vi "Confocal_0919 (1).vi"() -> ()   [LabVIEW 2017]
uses:
  <vilib>/Math Plots/2D Math Plots/XY Plot Matrix/XY Plot Matrix XCtrl/XY Plot Matrix.xctl
  Public/Documents/SIToolkit/LabVIEW/ExamplesXX_4_3_1_4/Spectroscopy Applications/GlobalCamOpen.vi
  Public/Documents/SIToolkit/LabVIEW/ExamplesXX_4_3_1_4/Spectroscopy Applications/GlobalInitializeFlag.vi
  Public/Documents/SIToolkit/LabVIEW/ExamplesXX_4_3_1_4/Spectroscopy Applications/GlobalTimingMode.vi
  Public/Documents/SIToolkit/LabVIEW/ExamplesXX_4_3_1_4/Spectroscopy Applications/GlobalFramesToStr.vi
  Public/Documents/SIToolkit/LabVIEW/ExamplesXX_4_3_1_4/Spectroscopy Applications/GlobalAcquireFocusFlag.vi
  Public/Documents/SIToolkit/LabVIEW/ExamplesXX_4_3_1_4/Spectroscopy Applications/GlobalExposure.vi
  <vilib>/Math Plots/2D Math Plots/XY Plot Matrix/XY Plot Matrix Datatype/XY Plot Matrix Datatype.lvclass
panel:
  out "Position 7":dbl[](array[numeric]) format="%.6f"
  out "Position 4":dbl[](array[numeric]) format="%.6f"
  in  "error PI Stage":errorcluster
  out "error out 2":errorcluster
  in  "Tab Control":T1(tab)
  in  "Focus/Acquire Mode":u32=1 min=1 max=5 step=1
  in  "Number of Frames to store":u32=1 min=1 step=1
  in  "Timing Mode":u32(ring)=1 items=["N/A", "Free Run/Timed", "Trigger First (PM only)", "Ext Sync/Strobed ", "Variable Exp (PM only)", "Flash Mode (PM only)"]
  out "Pixel Time":i32
  out "Bit Depth":i32
  out "ReadOut port":i32
  out "ADC Speed":i32
  in  "Set Experiment \nParameters, Initialize \nCamera/Controller":bool
  out "Read Temp.":dbl format="%.2f"
  in  "Set Temp.":dbl format="%.2f"
  in  "Exposure 2":dbl=0.2 format="%.2f"
  out "Controller Initialized":bool
  in  "error in":errorcluster
  out "error out":errorcluster
  in  "Power":dbl=10.0
  in  "Frequency":dbl=2810.0
  in  "Release Camera":bool
  out "Position 6":dbl[](array[numeric]) format="%.6f"
  out "Conn. Axis 5":string[](array[string])
  out "error out 3":errorcluster
  in  "stop":bool
  out "Read Frequency":dbl
  in  "Initial Frequency":dbl=2820.0
  in  "Final Frequency":dbl=2890.0
  in  "Step Size":dbl=3.0
  in  "OK Button 3":bool
  out "XY Plot Matrix":refnum<class "XY Plot Matrix Datatype.lvclass">[](xcontrol)
  out "history":dbl[][](array[numeric])
  in  "Number of Scans":i32
  out "COM Error":bool
  out "Camera Opened":bool
  out "Scan":i32
  in  "Number of Steps Left":dbl=5.0 format="%#_13g"
  in  "OK Button 5":bool
  in  "Step Size (microns)":dbl[](array[numeric])=[0.01]
  out "XY Plot Matrix":refnum<class "XY Plot Matrix Datatype.lvclass">[](xcontrol)
  in  "Number of Steps Down":dbl=5.0 format="%#_13g"
  out "Position":dbl[](array[numeric]) format="%.6f"
  out "Position 3":dbl[](array[numeric]) format="%.6f"
  in  "stop 2":bool
  out "Line Number":i32
  out "Position 2":dbl[](array[numeric]) format="%.6f"
  in  "?":bool
  out "Position 5":dbl[](array[numeric]) format="%.6f"
  in  "Step Size (microns) Y":dbl[](array[numeric])=[0.01]
  in  "Step Size (microns) X":dbl[](array[numeric])=[0.01]
  out "Position 8":dbl[](array[numeric]) format="%.6f"
  in  "?":bool
  in  "OK Button 4":bool
  in  "Frequency":dbl=2820.0
  out "XY Plot Matrix 2":refnum<class "XY Plot Matrix Datatype.lvclass">[](xcontrol) caption="XY Plot Matrix"
  out "history 2":dbl[][](array[numeric])
  in  "Points":i32=40
  in  "number of scans":i32=20
  out "Scan #":i32
  out "Point #":i32
  out "Acquire Graph":sgl[](graph)
  out "Collecting Data":bool
  in  "Full File Name for Acqure":path
  in  "OK Button":bool
  # "The following are read \nfrom camera after setting\nvalues to left.\n-1 value means item is not \nsupported by camera."
  # "Stage position on connection."
  # "Be sure to put in a full file name below before starting."
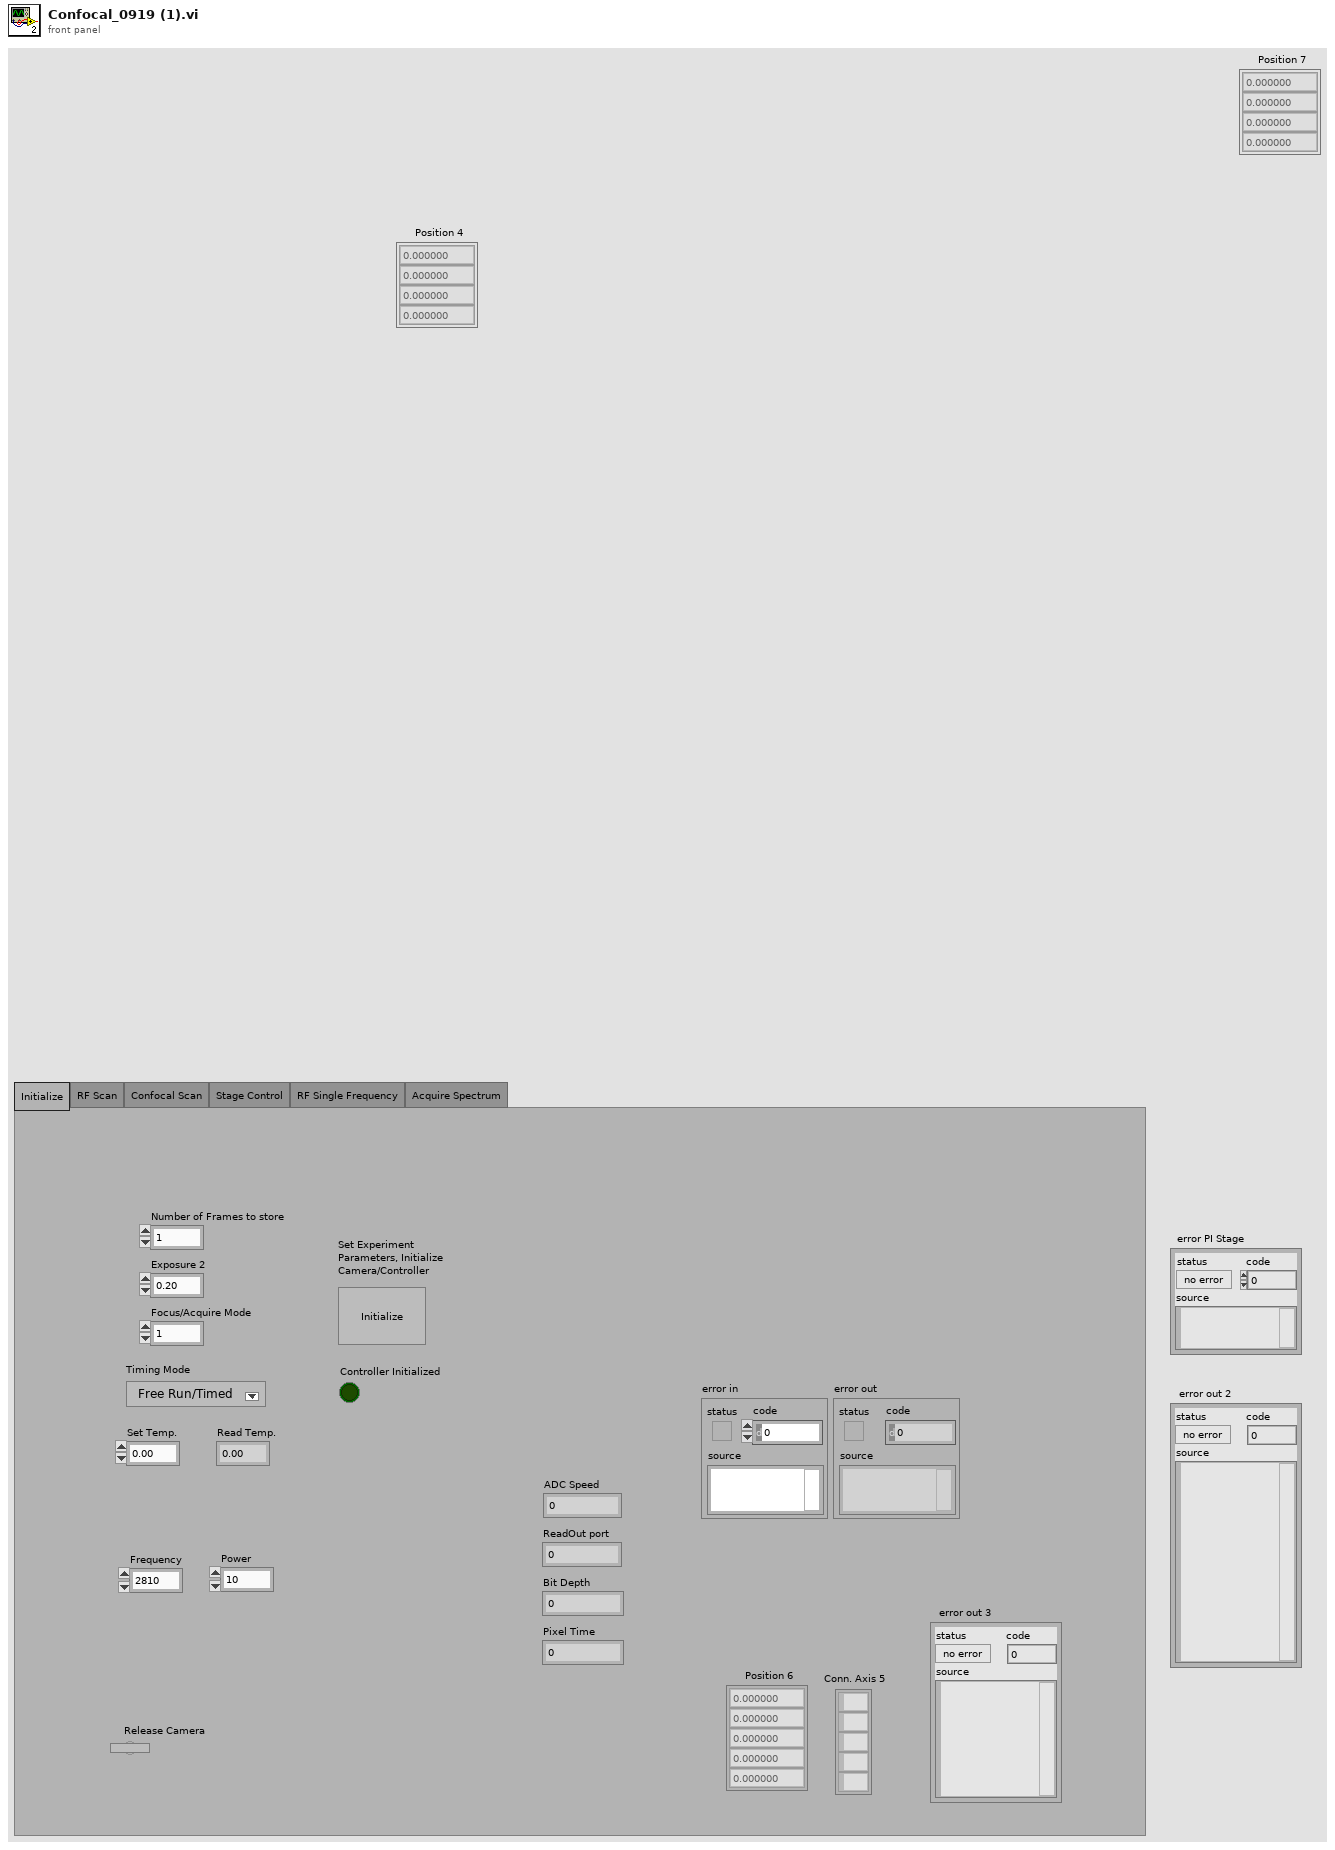
[diagram p1: front panel]
types:
  T1 = enum32{"Initialize", "RF Scan", "Confocal Scan", "Stage Control", "RF Single Frequency", "Acquire Spectrum"}
  T2 = cluster{"X start":u32, "X end":u32, "X Binning/Grouping":u32, "Y start":u32, "Y end":u32, "Y Binning/Grouping":u32}
  T3 = cluster{"Host address/name":string, "Port":i32, "Board":i32, "TCP/IP Search?":bool}
  T4 = cluster{"Camera Handle":u32, "Pulser Handle":u32, "File Handle":u32, "Display Handle":u32, "Image Handle":u32}
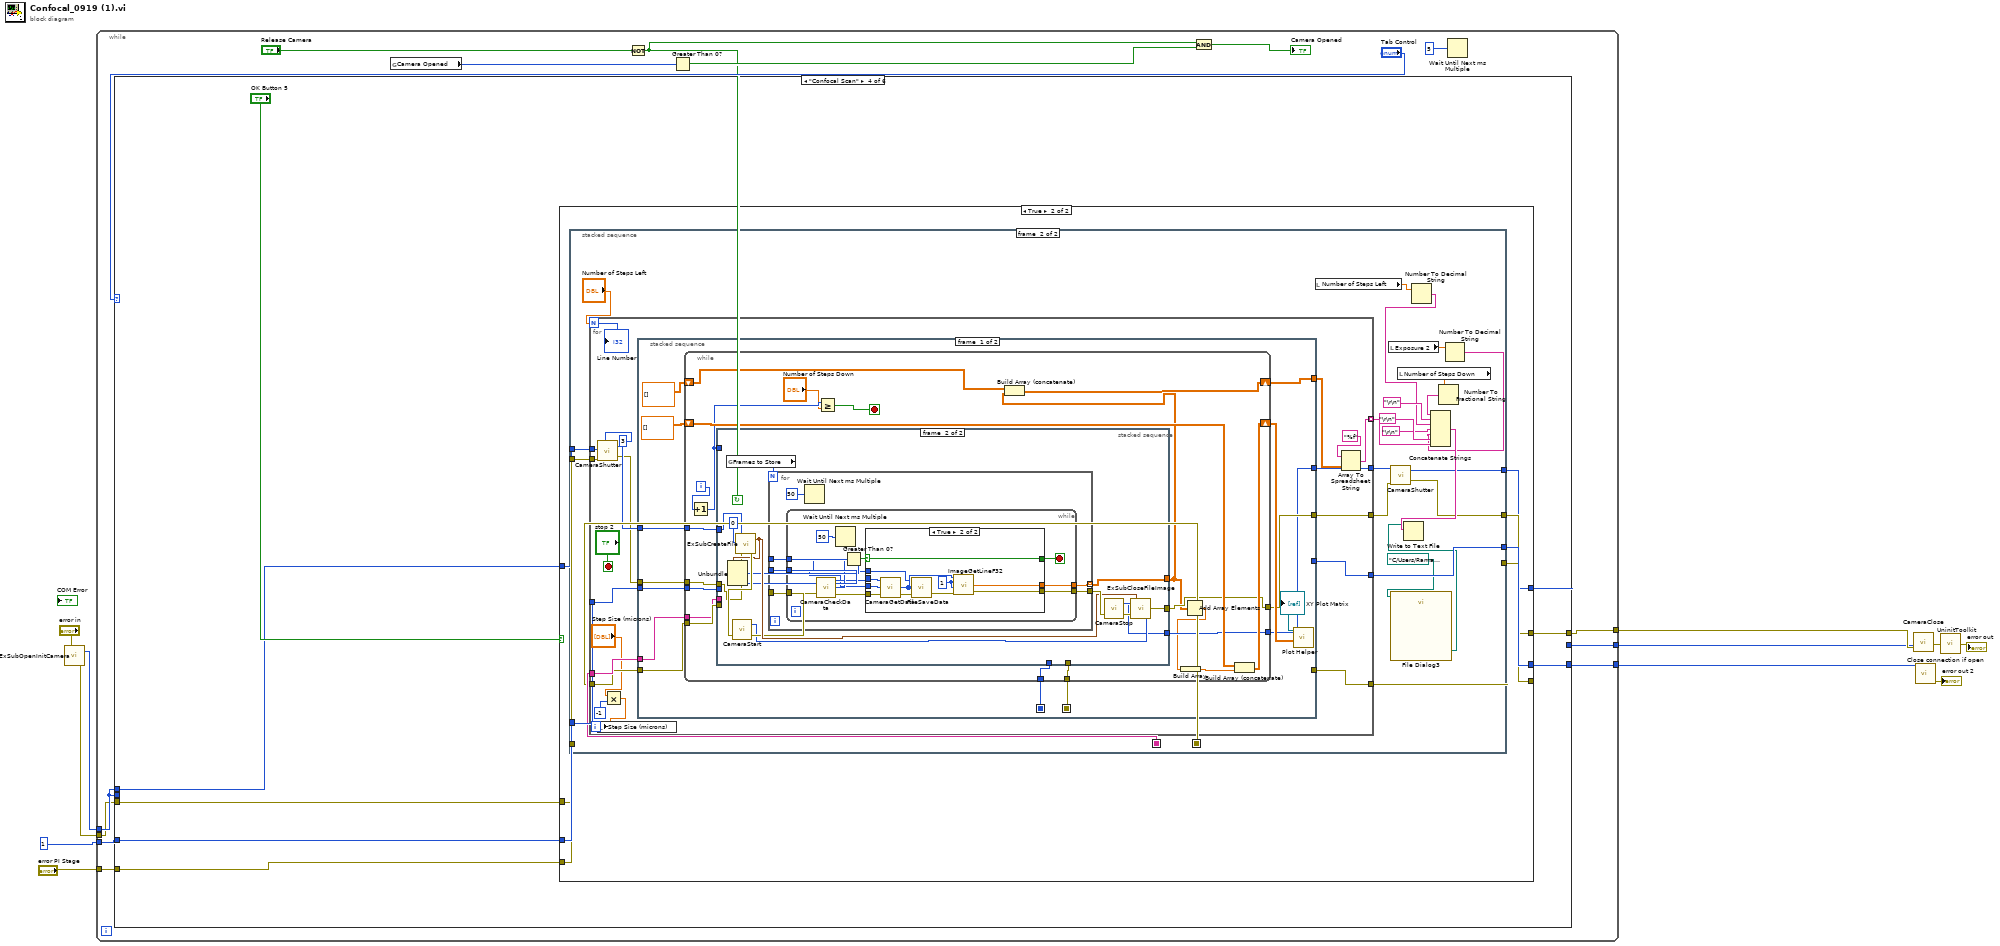
[diagram p0: block diagram]
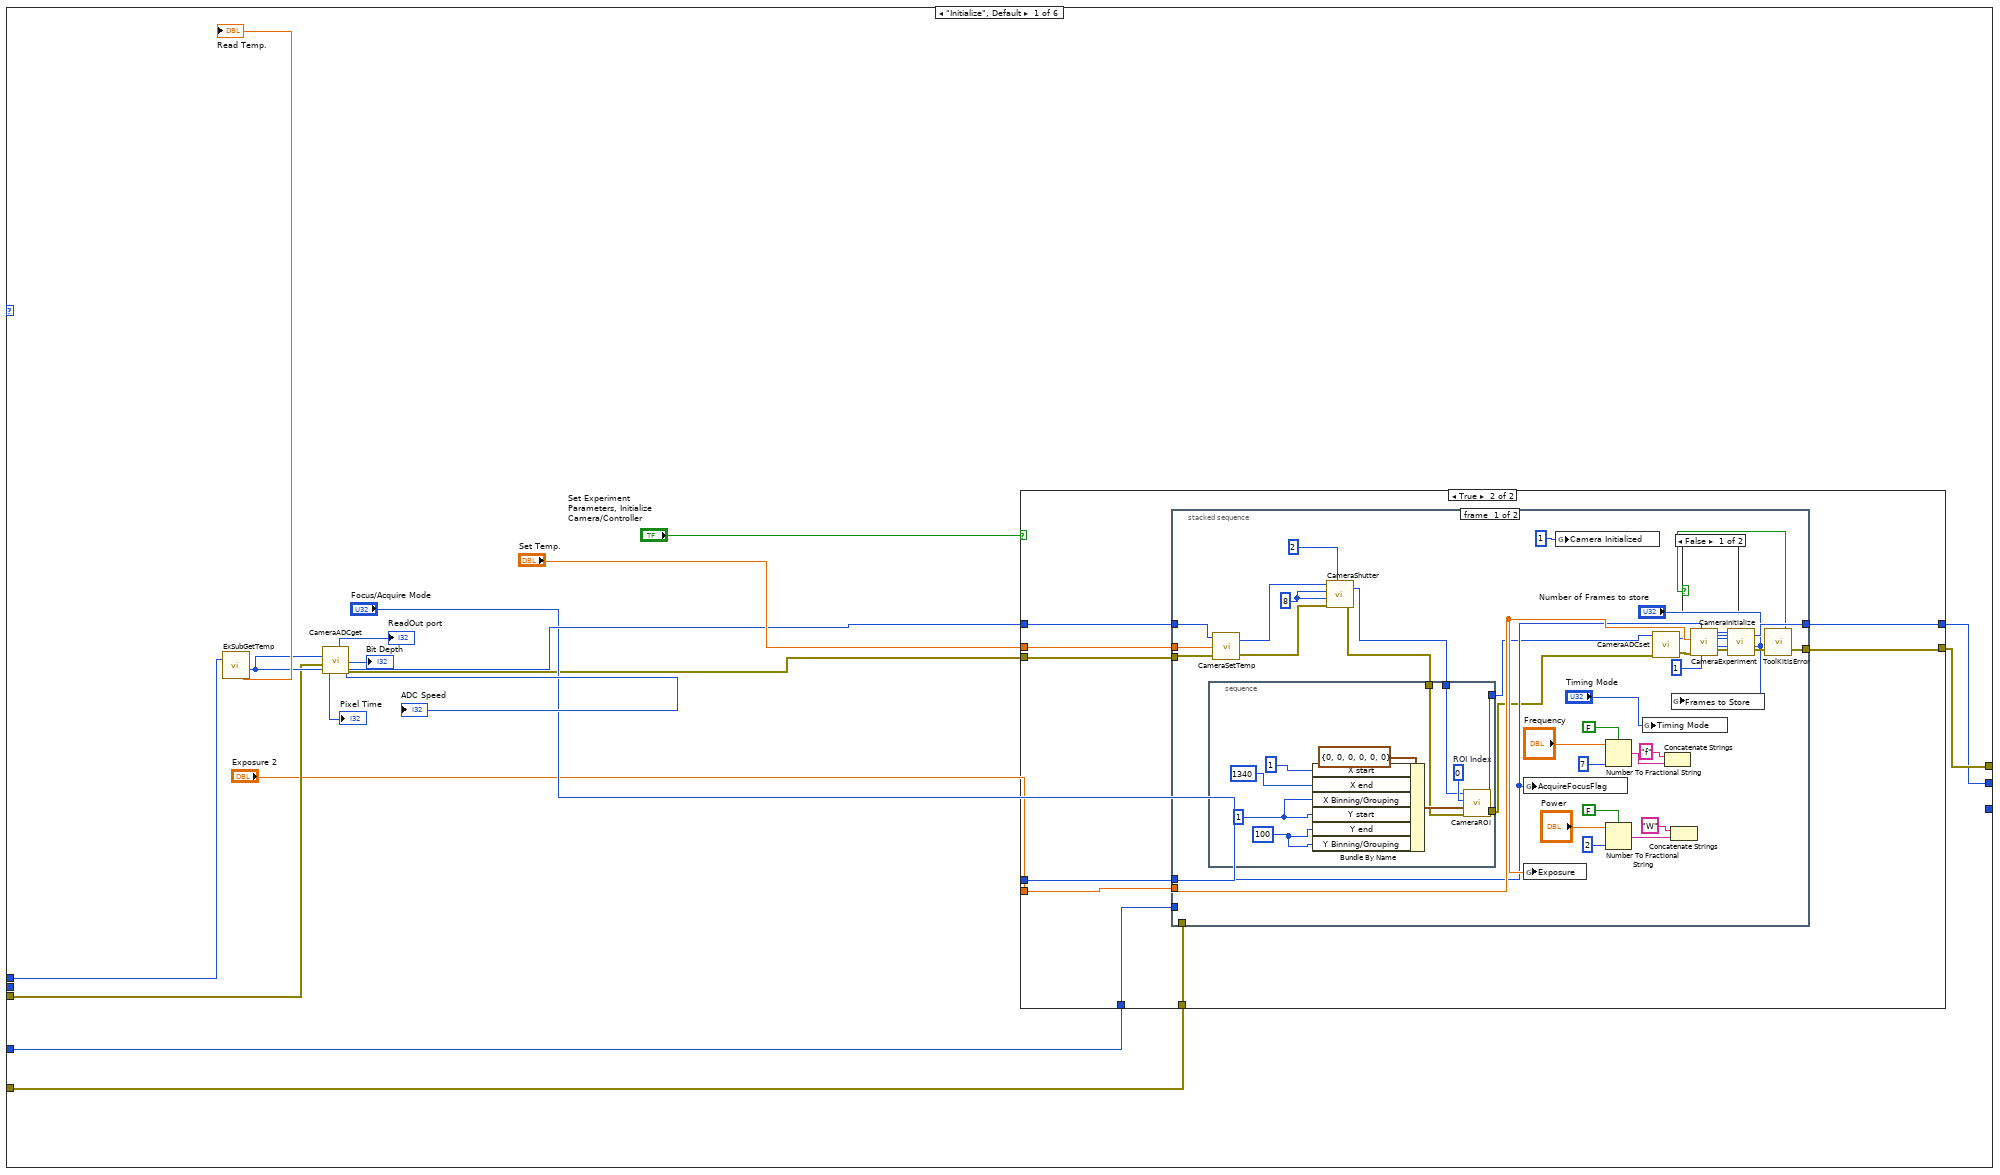
[diagram p2: hidden frame]
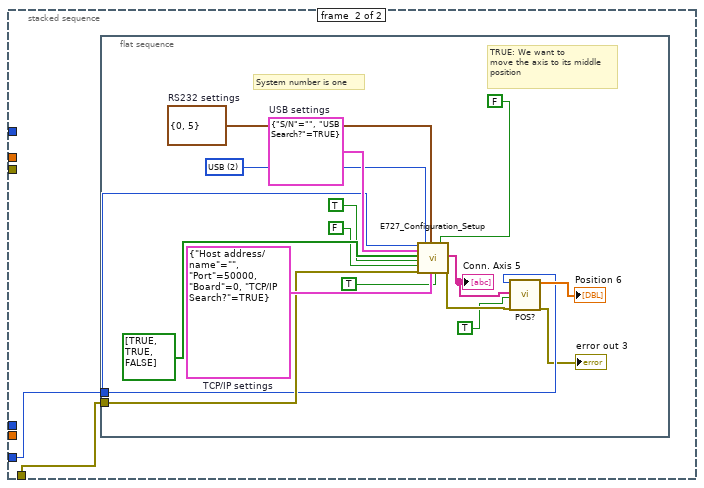
[diagram p5: hidden frame]
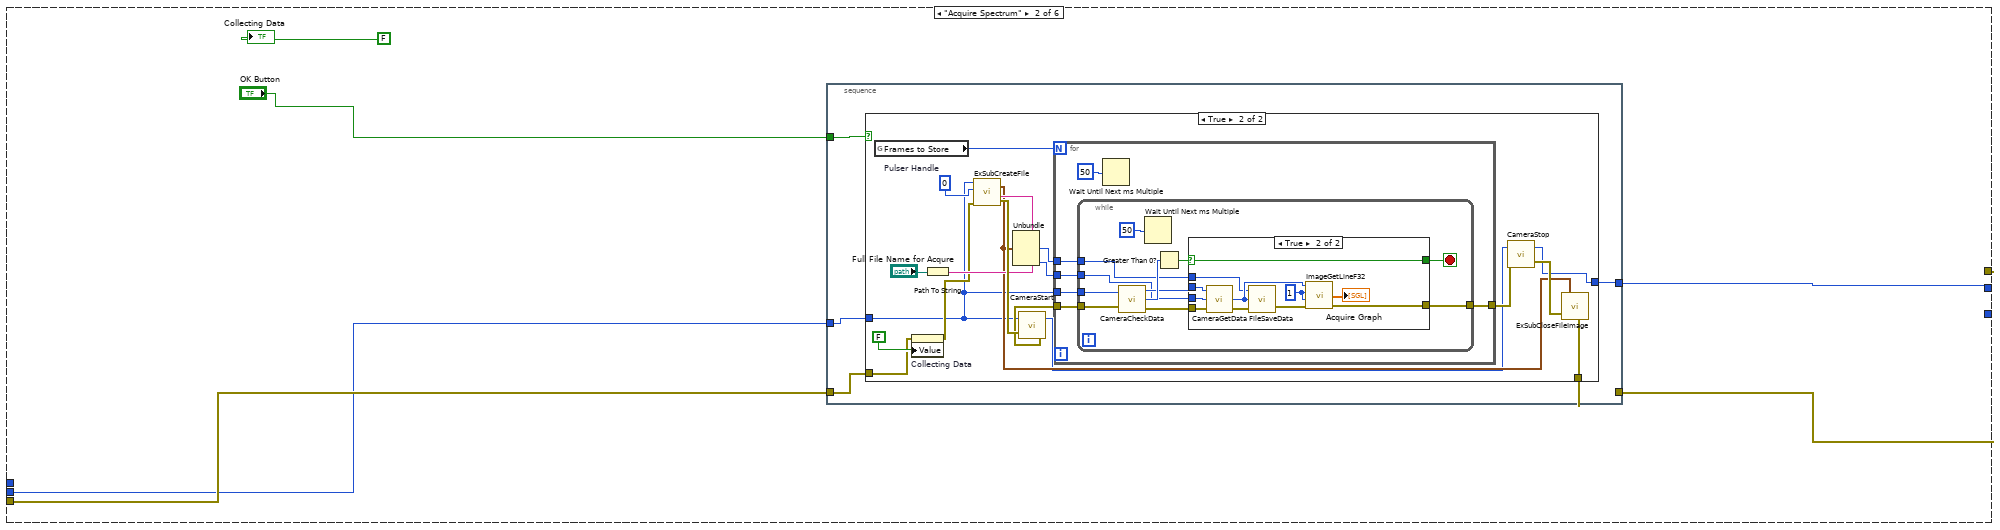
[diagram p6: hidden frame]
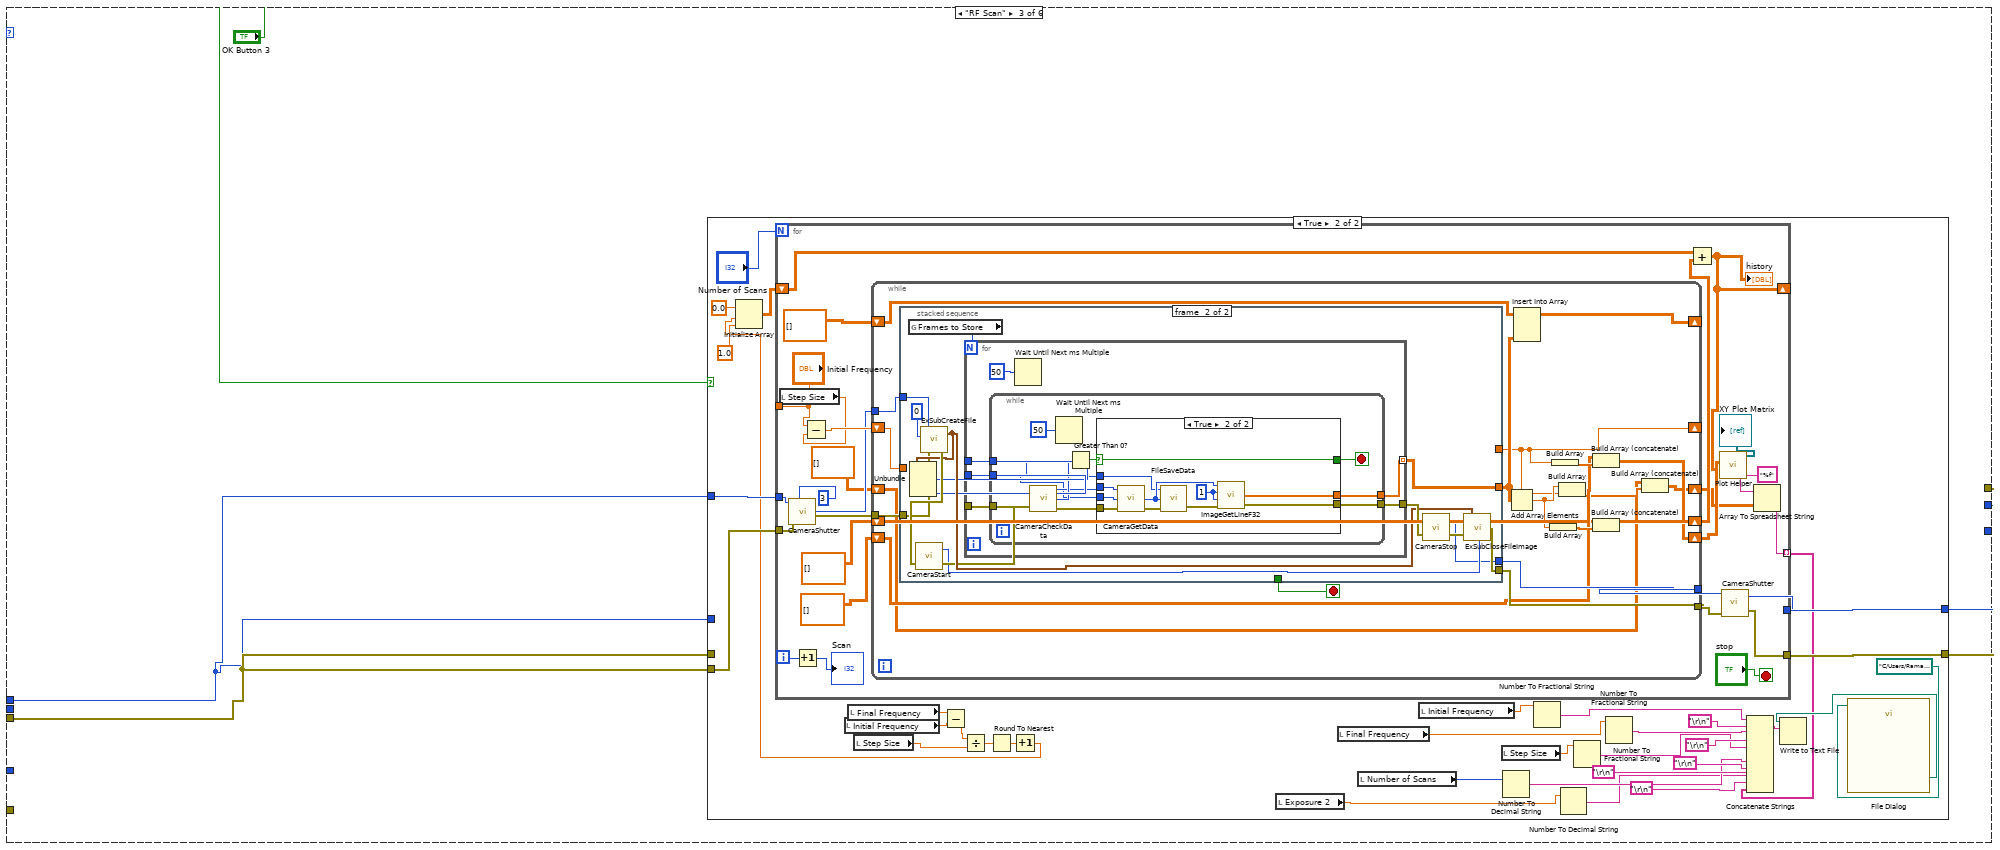
[diagram p9: hidden frame]
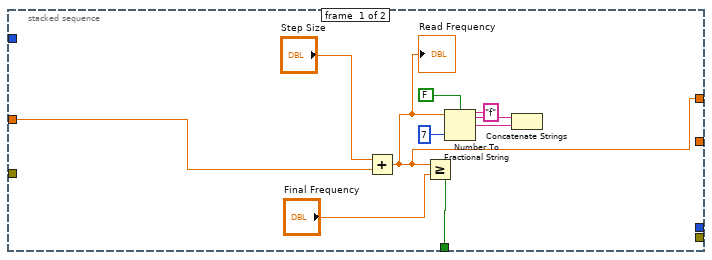
[diagram p11: hidden frame]
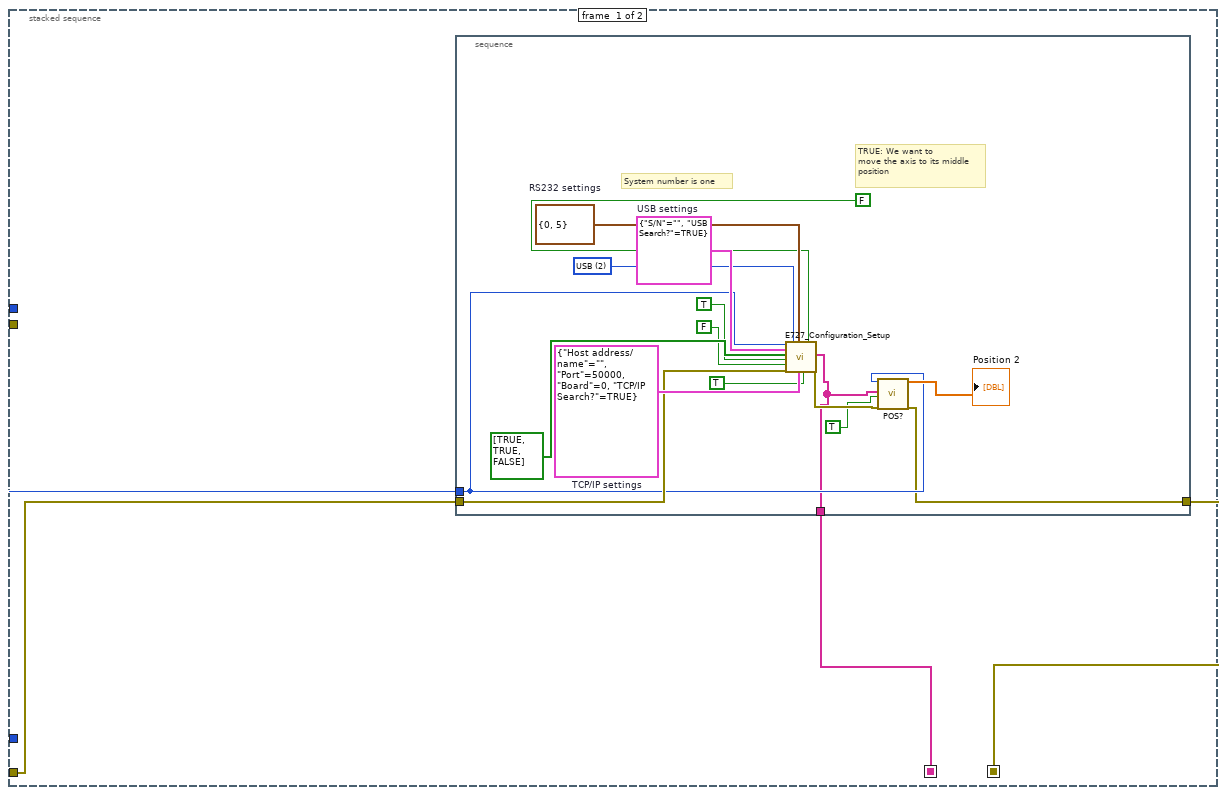
[diagram p14: hidden frame]
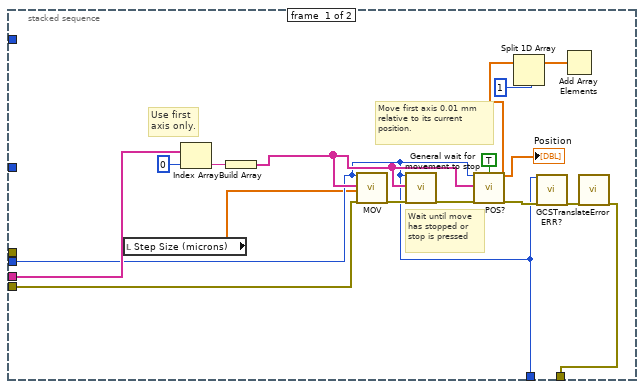
[diagram p15: hidden frame]
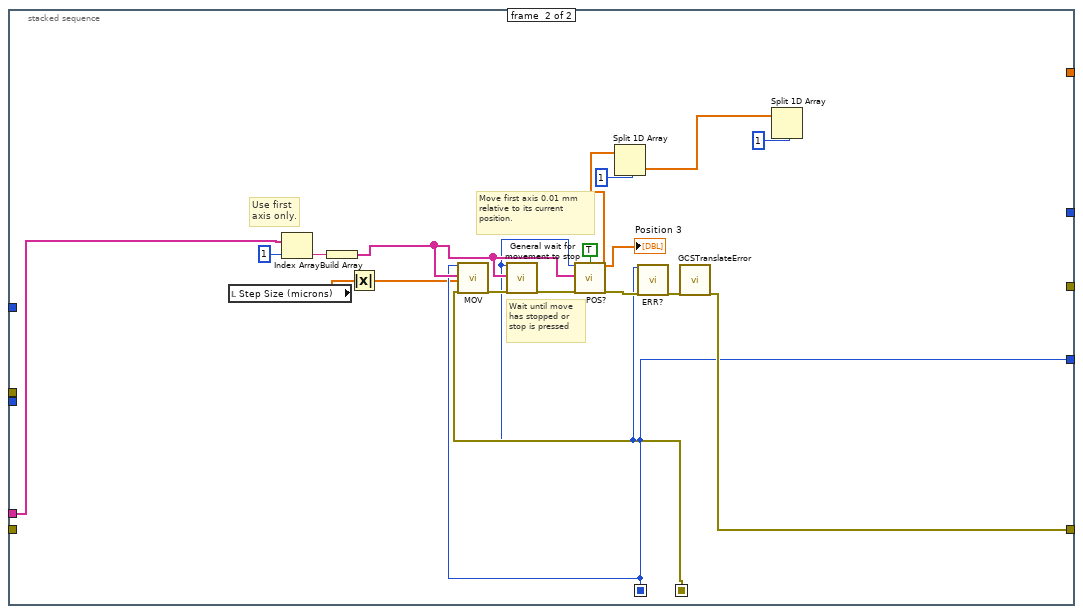
[diagram p17: hidden frame]
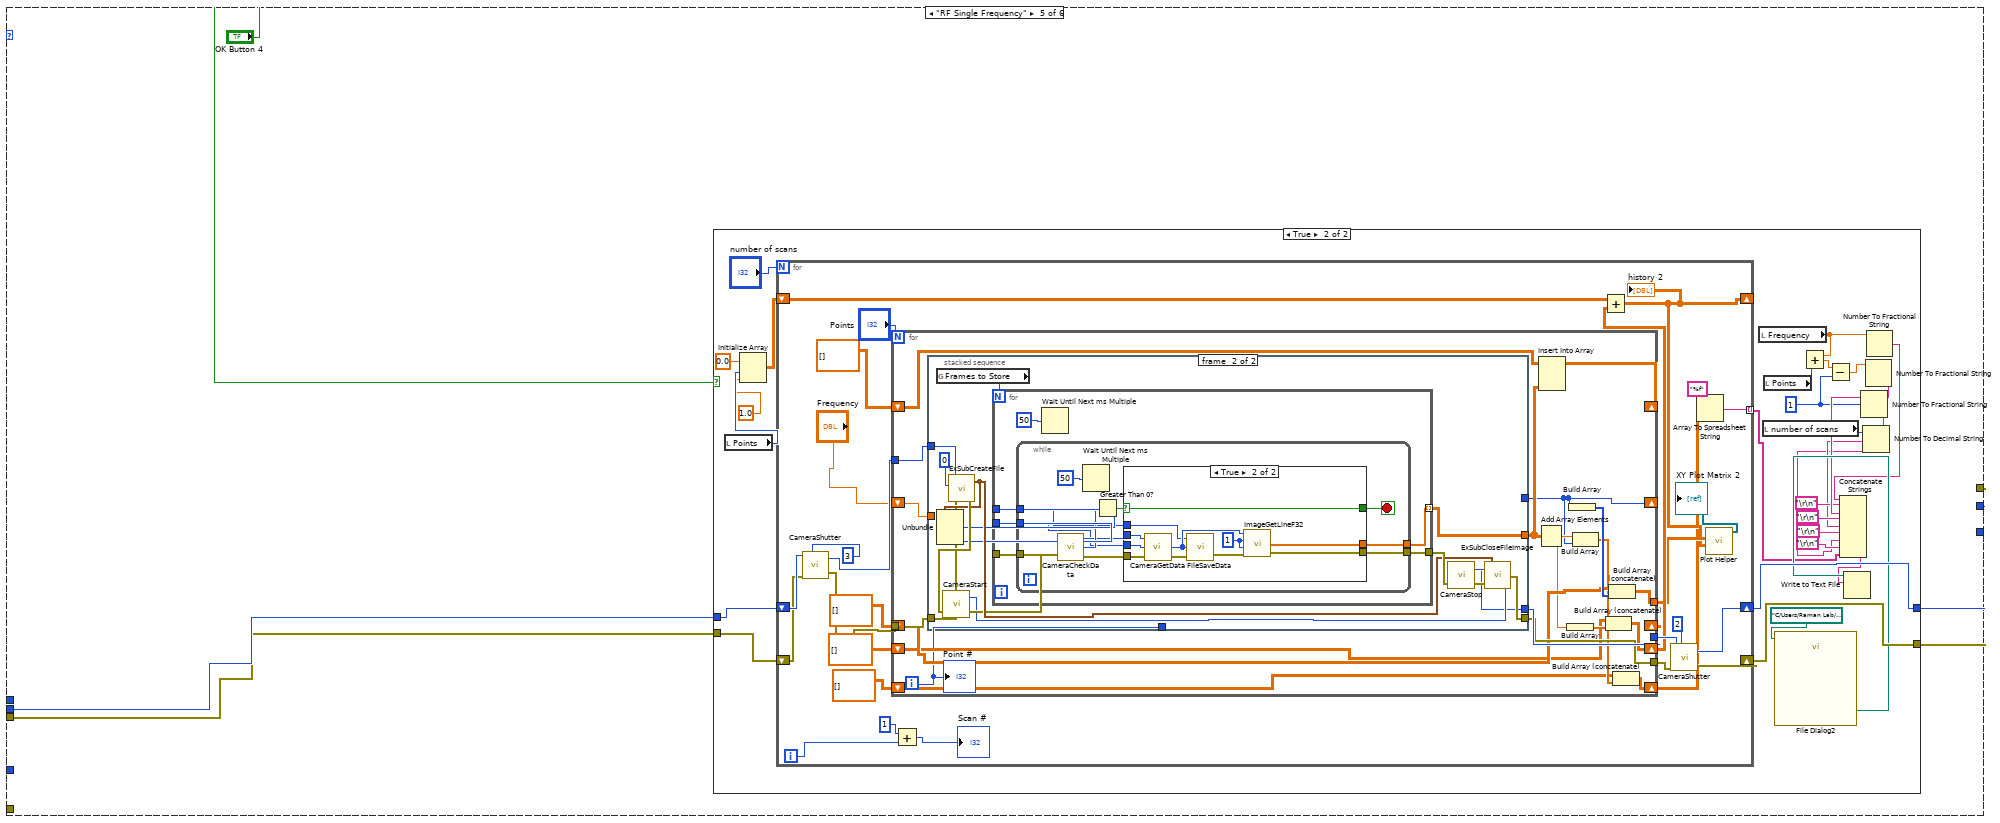
[diagram p18: hidden frame]
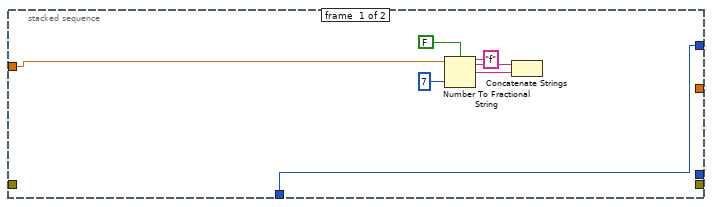
[diagram p20: hidden frame]
diagram:
  n1 = call "ExSubOpenInitCamera.vi"("error in (no error)"="error in") -> ("Camera Handle"=w10:u32, "error out"=w9:errorcluster)
  n2 = while {
    tunnel: w10 -> [w19]
    tunnel: w9 -> [w18]
    tunnel: [w17] -> w8
    tunnel: [w15] -> w5
    tunnel: "error PI Stage" -> [w14]
    tunnel: 1 -> [w12]
    tunnel: [w13] -> w1
    stop <- w16 continue-if-true
    n3 = case shown="\"Confocal Scan\"" "Tab Control" {
      tunnel: w19 -> [w34 _ w181 w323 _ _]
      tunnel: w19 -> [_ w123 _ _ w521 _]
      tunnel: w18 -> [w33 w124 w183 w324 w520 _]
      tunnel: [w28 w120 w182 w325 w519 _] -> w15
      tunnel: [w30 w121 w184 w326 w518 _] -> w17
      tunnel: w14 -> [w26 _ _ w328 _ w649]
      tunnel: w12 -> [w27 _ _ w330 _ w650]
      tunnel: [_ _ _ w329 _ _] -> w13
      frame "Initialize", Default {
        n4 = call "ExSubGetTemp.vi"("Camera Handle"=w34) -> ("Camera Handle"=w39:u32, "Temperature Real"=→"Read Temp.":dbl)  [unwired: 1 in, 1 out]
        n5 = call <userlib>:"CameraADCget.vi"("Camera handle"=w39, "error in (no error)"=w33) -> ("Bit Depth"=→"Bit Depth":i32, "Pixel Time"=→"Pixel Time":i32, "Readout Port"=→"ReadOut port":i32, "ADC Speed"=→"ADC Speed":i32, "error out"=w32:errorcluster)  [unwired: 3 out]
        n6 = case shown="True" "Set Experiment \nParameters, Initialize \nCamera/Controller" {
          tunnel: "Exposure 2" -> [_ w53]
          tunnel: "Set Temp." -> [_ w54]
          tunnel: w39 -> [w46 w55]
          tunnel: [w46 w52] -> w28
          tunnel: "Focus/Acquire Mode" -> [_ w51]
          tunnel: w32 -> [w45 w50]
          tunnel: [w45 w49] -> w30
          tunnel: w27 -> [_ w48]
          tunnel: w26 -> [_ w47]
          frame False {
          }
          frame True {
            n7 = stacked-sequence {
              tunnel: w55 -> [w90 _]
              tunnel: w54 -> [w89 _]
              tunnel: w53 -> [w88 _]
              tunnel: [w87 _] -> w52
              tunnel: w51 -> [w86 _]
              tunnel: w50 -> [w85 _]
              tunnel: [w84 _] -> w49
              tunnel: w48 -> [_ w102]
              tunnel: w47 -> [_ w103]
              frame #0 {
                w56 = 8
                n8 = call <userlib>:"CameraSetTemp.vi"("error in (no error)"=w85, "Temperature"=w89, "Camera Handle"=w90) -> ("error out"=w59:errorcluster, "Camera Handle"=w61:u32)
                n9 = call <userlib>:"CameraShutter.vi"("Camera Handle"=w61, "Shutter Comp Time: Pre Open"=w56, "Shutter Comp Time: Post Open"=w56, "error in"=w59, "Shutter State"=2) -> ("Camera Handle"=w60:u32, "error out"=w58:errorcluster)
                n10 = stacked-sequence {
                  tunnel: [w98] -> w63
                  tunnel: w60 -> [w95]
                  tunnel: w58 -> [w94]
                  tunnel: [w93] -> w62
                  frame #0 {
                    w97 = 100
                    w91 = 1
                    w100 = u32 0  # ROI Index
                    n11 = Bundle By Name(cluster=T2 {"X start"=0, "X end"=0, "X Binning/Grouping"=0, "Y start"=0, "Y end"=0, "Y Binning/Grouping"=0} ("ROI Params"), "X start"=1, "X end"=1340, "X Binning/Grouping"=w91, "Y start"=w91, "Y end"=w97, "Y Binning/Grouping"=w97) -> (w101:T2)
                    n12 = call <userlib>:"CameraROI.vi"("error in"=w94, "ROI Params"=w101, "ROI Index"=w100, "Camera Handle"=w95) -> ("error out"=w93:errorcluster, "Camera Handle"=w98:u32)
                  }
                }
                n13 = global write "GlobalAcquireFocusFlag.vi" "AcquireFocusFlag"(w86) -> ()
                n14 = global write "GlobalExposure.vi" "Exposure"(w88) -> ()
                n15 = global write "GlobalInitializeFlag.vi" "Camera Initialized"(1) -> ()
                n16 = Number To Fractional String(use system decimal point (T)=FALSE, number="Frequency", precision (6)=7) -> (F-format string=w65:string)  [unwired: 1 in]
                n17 = Number To Fractional String(use system decimal point (T)=FALSE, number="Power", precision (6)=2) -> (F-format string=w72:string)  [unwired: 1 in]
                n18 = global write "GlobalTimingMode.vi" "Timing Mode"("Timing Mode") -> ()
                n19 = call <userlib>:"CameraADCset.vi"("error in (no error)"=w62, "Camera Handle"=w63) -> ("error out"=w80:errorcluster, "Camera Handle"=w79:u32)  [unwired: 4 in]
                n20 = Concatenate Strings("f", w65) -> ()  [unwired: 1 out]
                n21 = Concatenate Strings("W", w72) -> ()  [unwired: 1 out]
                n22 = global write "GlobalFramesToStr.vi" "Frames to Store"("Number of Frames to store") -> ()
                n23 = call <userlib>:"CameraExperiment.vi"("Number of Accumulations"=1, "Acquire / Focus Flag"=w86, "error in"=w80, "Number of Images"="Number of Frames to store", "Exposure (sec)"=w88, "Camera Handle"=w79) -> ("error out"=w78:errorcluster, "Camera Handle"=w77:u32)
                n24 = call <userlib>:"CameraInitialize.vi"("error in"=w78, "Camera Handle"=w77) -> ("error out"=w75:errorcluster, "Camera Handle"=w87:u32)
                n25 = call <userlib>:"ToolKitIsError.vi"("error in"=w75) -> ("error out"=w84:errorcluster, "Error Flag"=w76:bool)  [unwired: 1 in]
                n26 = case shown="False" w76 {
                  frame False {
                  }
                  frame True {
                  }
                }
              }
              frame #1 {
                n27 = flat-sequence {
                  tunnel: w103 -> [w107]
                  tunnel: w102 -> [w106]
                  frame #0 {
                    w119 = cluster{"S/N":string, "USB Search?":bool} {"S/N"="", "USB Search?"=TRUE}  # USB settings
                    w115 = u16 2 items=["RS232", "TCP/IP", "USB"] ("Interface")
                    w114 = cluster{"Portnumber":i32, "Baudrate":u16} {"Portnumber"=0, "Baudrate"=5}  # RS232 settings
                    w113 = T3 {"Host address/name"="", "Port"=50000, "Board"=0, "TCP/IP Search?"=TRUE}  # TCP/IP settings
                    # "TRUE: We want to\nmove the axis to its middle\nposition"
                    # "System number is one"
                    n28 = call "E727_Configuration_Setup.vi"("System no."=w106, "USB settings"=w119, "Are stages connected?"=bool[] [TRUE, TRUE, FALSE], "Change servo status to ON?"=TRUE ("Use dialog to define\nconnected stages?"), "Perform autozero?"=FALSE ("Use dialog to define\nconnected stages?"), "error in"=w107, "Interface"=w115, "RS232 settings"=w114, "TCP/IP settings"=w113, "Stop wave generator\noutput (if any)"=TRUE ("All axes?"), "Move to middle?"=FALSE) -> ("All conn. axes"=w105:string[], "error out"=w109:errorcluster)  [unwired: 3 in, 4 out]
                    "Conn. Axis 5" <- w105
                    n29 = call "POS?.vi"("System no."=w106, "Axes to query"=w105, "All axes?"=TRUE, "error in"=w109) -> ("Position"=→"Position 6":dbl[], "error out"=→"error out 3":errorcluster)  [unwired: 1 in, 13 out]
                  }
                }
              }
            }
          }
        }
        n30 = global read "GlobalInitializeFlag.vi" "Camera Initialized"() -> (w42:u32)
        n31 = Greater Than 0?(x=w42) -> (x > 0?=→"Controller Initialized":bool)
      }
      frame "Acquire Spectrum" {
        n32 = stacked-sequence {
          tunnel: [w127] -> w121
          tunnel: [w128] -> w120
          tunnel: w124 -> [w130]
          tunnel: "OK Button" -> [w129]
          tunnel: w123 -> [w126]
          frame #0 {
            n33 = case shown="True" w129 {
              tunnel: [w131 w143] -> w128
              tunnel: [w132 w135] -> w127
              tunnel: w130 -> [w132 w134]
              tunnel: w126 -> [w131 w133]
              frame False {
              }
              frame True {
                w137 = u32 0  # Pulser Handle
                n34 = global read "GlobalFramesToStr.vi" "Frames to Store"() -> (w146:u32)
                n35 = property on="Collecting Data" class="Bool (strict)"(error in=w134, "Value"=FALSE) -> (error out=w145:errorcluster)  [unwired: 1 in, 1 out]
                n36 = Path To String(path="Full File Name for Acqure") -> (string=w148:string)
                n37 = call "ExSubCreateFile.vi"("error in (no error)"=w145, "File and Display Name"=w148, "Pulser Handle"=w137, "Camera Handle"=w133) -> ("error out"=w150:errorcluster, "Handles Out"=w141:T4)
                n38 = Unbundle(w141) -> ("File Handle"=w136:u32, "Image Handle"=w139:u32)  [unwired: 3 out]
                n39 = call <userlib>:"CameraStart.vi"("error in"=w150, "Camera Handle"=w133) -> ("error out"=w140:errorcluster, "Camera Handle"=w138:u32)
                n40 = for {
                  N: w146 -> [_]
                  tunnel: w133 -> [w155]
                  tunnel: w140 -> [w154]
                  tunnel: [w153] -> w142
                  tunnel: w136 -> [w152]
                  tunnel: w139 -> [w151]
                  n41 = while {
                    tunnel: [w162] -> w153
                    tunnel: w155 -> [w160]
                    tunnel: w154 -> [w159]
                    tunnel: w152 -> [w158]
                    tunnel: w151 -> [w157]
                    stop <- w163 stop-if-true
                    n42 = call <userlib>:"CameraCheckData.vi"("Camera Handle"=w160, "error in"=w159) -> ("Camera Handle"=w165:u32, "Number Of Frames Available"=w167:i32, "error out"=w164:errorcluster)
                    n43 = Wait Until Next ms Multiple(millisecond multiple=u32 50) -> ()  [unwired: 1 out]
                    n44 = Greater Than 0?(x=w167) -> (x > 0?=w166:bool)
                    n45 = case shown="True" w166 {
                      selector: w166 -> [w168 w178]
                      tunnel: w165 -> [_ w180]
                      tunnel: w164 -> [w169 w179]
                      tunnel: [w168 w178] -> w163
                      tunnel: [w169 w173] -> w162
                      tunnel: w158 -> [_ w171]
                      tunnel: w157 -> [_ w170]
                      frame False {
                      }
                      frame True {
                        w174 = 1
                        n46 = call <userlib>:"CameraGetData.vi"("error in"=w179, "Image/Data Handle"=w170, "Camera Handle"=w180) -> ("error out"=w177:errorcluster, "Image/Data Handle"=w175:u32)  [unwired: 1 out]
                        n47 = call <userlib>:"FileSaveData.vi"("error in"=w177, "Image Handle"=w175, "File Handle"=w171) -> ("error out"=w176:errorcluster)  [unwired: 1 out]
                        n48 = call <userlib>:"ImageGetLineF32.vi"("error in"=w176, "Z Position"=w174, "Y Position"=w174, "Data Handle"=w175) -> ("error out"=w173:errorcluster, "Array F32"=→"Acquire Graph":sgl[])  [unwired: 1 out]
                      }
                    }
                  }
                  n49 = Wait Until Next ms Multiple(millisecond multiple=u32 50) -> ()  [unwired: 1 out]
                }
                n50 = call <userlib>:"CameraStop.vi"("error in"=w142, "Camera Handle"=w138) -> ("error out"=w147:errorcluster, "Camera Handle"=w143:u32)
                n51 = call "ExSubCloseFileImage.vi"("error in (no error)"=w147, "Handles In"=w141) -> ("error out"=w135:errorcluster)
              }
            }
          }
        }
        "Collecting Data" <- FALSE
      }
      frame "RF Scan" {
        n52 = case shown="True" "OK Button 3" {
          tunnel: w181 -> [w187 _]
          tunnel: w183 -> [w186 _]
          tunnel: [w187 w207] -> w182
          tunnel: [w186 w206] -> w184
          tunnel: w181 -> [_ w209]
          tunnel: w183 -> [_ w208]
          frame False {
          }
          frame True {
            n53 = local read "Initial Frequency"() -> (w197:dbl)
            n54 = local read "Final Frequency"() -> (w198:dbl)
            n55 = local read "Step Size"() -> (w195:dbl)
            n56 = Subtract(x=w198, y=w197) -> (x-y=w196:dbl)
            n57 = Divide(x=w196, y=w195) -> (x/y=w194:dbl)
            n58 = Round To Nearest(number=w194) -> (nearest integer value=w193:dbl)
            n59 = Increment(x=w193) -> (x+1=w192:dbl)
            n60 = Initialize Array(0.0, w192, 1.0) -> (w200:dbl[][])
            n61 = for {
              N: "Number of Scans" -> [_]
              tunnel: w209 -> [w242]
              tunnel: w208 -> [w241]
              tunnel: [w237] -> w207
              tunnel: [w236] -> w206
              shift-right: [w227] -> _
              shift-left: w200 -> [w231]
              tunnel: ["Initial Frequency"] -> _
              tunnel: [w226] -> w191 mode=indexing
              i -> [w233]
              stop <- "stop" stop-if-true
              n62 = local read "Step Size"() -> (w243:dbl)
              n63 = call <userlib>:"CameraShutter.vi"("Camera Handle"=w242, "error in"=w241, "Shutter State"=3) -> ("Camera Handle"=w238:u32, "error out"=w239:errorcluster)  [unwired: 2 in]
              n64 = Increment(x=w233) -> (x+1=→"Scan":i32)
              n65 = Subtract(x="Initial Frequency", y=w243) -> (x-y=w248:dbl)
              n66 = while {
                shift-right: [w253] -> _
                shift-left: w248 -> [w266]
                tunnel: [w268] -> w245
                tunnel: [w267] -> w244
                shift-right: [w262] -> _
                shift-left: dbl[][] [] -> [w263]
                tunnel: w239 -> [w265]
                tunnel: w238 -> [w264]
                shift-right: [w255] -> w229
                shift-left: dbl[][] [] -> [w259]
                shift-right: [w256] -> w230
                shift-left: dbl[][] [] -> [w257]
                shift-right: [w250] -> w223
                shift-left: dbl[][] [] -> [w251]
                stop <- w249 stop-if-true
                n67 = stacked-sequence {
                  tunnel: w266 -> [w272 _]
                  tunnel: [_ w281] -> w268
                  tunnel: [_ w282] -> w267
                  tunnel: [w271 _] -> w253
                  tunnel: [_ w280] -> w258
                  tunnel: w265 -> [_ w279]
                  tunnel: w264 -> [_ w278]
                  tunnel: [w269 _] -> w249
                  frame #0 {
                    n68 = Add(x="Step Size", y=w272) -> (x+y=w271:dbl)
                    "Read Frequency" <- w271
                    n69 = Greater Or Equal?(x=w271, y="Final Frequency") -> (x >= y?=w269:bool)
                    n70 = Number To Fractional String(use system decimal point (T)=FALSE, number=w271, precision (6)=7) -> (F-format string=w277:string)  [unwired: 1 in]
                    n71 = Concatenate Strings("f", w277) -> ()  [unwired: 1 out]
                  }
                  frame #1 {
                    n72 = global read "GlobalFramesToStr.vi" "Frames to Store"() -> (w290:u32)
                    n73 = call "ExSubCreateFile.vi"("error in (no error)"=w279, "Pulser Handle"=u32 0, "Camera Handle"=w278) -> ("error out"=w292:errorcluster, "Handles Out"=w288:T4)  [unwired: 1 in]
                    n74 = Unbundle(w288) -> ("File Handle"=w283:u32, "Image Handle"=w286:u32)  [unwired: 3 out]
                    n75 = call <userlib>:"CameraStart.vi"("error in"=w292) -> ("error out"=w287:errorcluster, "Camera Handle"=w285:u32)  [unwired: 1 in]
                    n76 = for {
                      N: w290 -> [_]
                      tunnel: w287 -> [w297]
                      tunnel: [w296] -> w289
                      tunnel: w283 -> [w295]
                      tunnel: w286 -> [w294]
                      tunnel: [w293] -> w280 mode=indexing
                      n77 = while {
                        tunnel: [w304] -> w296
                        tunnel: w297 -> [w302]
                        tunnel: w295 -> [w301]
                        tunnel: w294 -> [w300]
                        tunnel: [w299] -> w293
                        stop <- w305 stop-if-true
                        n78 = call <userlib>:"CameraCheckData.vi"("error in"=w302) -> ("Camera Handle"=w307:u32, "Number Of Frames Available"=w309:i32, "error out"=w306:errorcluster)  [unwired: 1 in]
                        n79 = Wait Until Next ms Multiple(millisecond multiple=u32 50) -> ()  [unwired: 1 out]
                        n80 = Greater Than 0?(x=w309) -> (x > 0?=w308:bool)
                        n81 = case shown="True" w308 {
                          selector: w308 -> [w310 w320]
                          tunnel: w307 -> [_ w322]
                          tunnel: w306 -> [w311 w321]
                          tunnel: [w310 w320] -> w305
                          tunnel: [w311 w315] -> w304
                          tunnel: w301 -> [_ w314]
                          tunnel: w300 -> [_ w313]
                          tunnel: [_ w312] -> w299
                          frame False {
                          }
                          frame True {
                            w316 = 1
                            n82 = call <userlib>:"CameraGetData.vi"("error in"=w321, "Image/Data Handle"=w313, "Camera Handle"=w322) -> ("error out"=w319:errorcluster, "Image/Data Handle"=w317:u32)  [unwired: 1 out]
                            n83 = call <userlib>:"FileSaveData.vi"("error in"=w319, "Image Handle"=w317, "File Handle"=w314) -> ("error out"=w318:errorcluster)  [unwired: 1 out]
                            n84 = call <userlib>:"ImageGetLineF32.vi"("error in"=w318, "Z Position"=w316, "Y Position"=w316, "Data Handle"=w317) -> ("error out"=w315:errorcluster, "Array F32"=w312:sgl[])  [unwired: 1 out]
                          }
                        }
                      }
                      n85 = Wait Until Next ms Multiple(millisecond multiple=u32 50) -> ()  [unwired: 1 out]
                    }
                    n86 = call <userlib>:"CameraStop.vi"("error in"=w289, "Camera Handle"=w285) -> ("error out"=w291:errorcluster, "Camera Handle"=w281:u32)
                    n87 = call "ExSubCloseFileImage.vi"("error in (no error)"=w291, "Handles In"=w288) -> ("error out"=w282:errorcluster)
                  }
                }
                n88 = Add Array Elements(numeric array=w258) -> (sum=w254:sgl)
                n89 = Insert Into Array(array=w263, new element=w258) -> (w262:dbl[][])  [unwired: 2 in]
                n90 = Build Array(w254) -> (w260:sgl[])
                n91 = Build Array(w253) -> (w261:dbl[])
                n92 = Build Array(w254, w253) -> (w252:dbl[])
                n93 = Build Array (concatenate)(w259, w261) -> (w255:dbl[][])
                n94 = Build Array (concatenate)(w257, w260) -> (w256:dbl[][])
                n95 = Build Array (concatenate)(w251, w252) -> (w250:dbl[][])
              }
              n96 = Add(x=w231, y=w230) -> (x+y=w227:dbl[][])
              "history" <- w227
              n97 = call <vilib>:"Plot Helper.vi"("y matrix"=w227, "x matrix"=w229) -> ("2D Plotmatrix Class Obj Array out"=→"XY Plot Matrix":refnum<class "XY Plot Matrix Datatype.lvclass">[])  [unwired: 2 in, 7 out]
              n98 = call <userlib>:"CameraShutter.vi"("Camera Handle"=w245, "error in"=w244) -> ("Camera Handle"=w237:u32, "error out"=w236:errorcluster)  [unwired: 3 in]
              n99 = Array To Spreadsheet String(array=w223, 3:"%f" ("format string")) -> (spreadsheet string=w226:string)  [unwired: 1 in]
            }
            n100 = local read "Exposure 2"() -> (w188:dbl)
            n101 = local read "Final Frequency"() -> (w204:dbl)
            n102 = local read "Number of Scans"() -> (w202:i32)
            n103 = local read "Initial Frequency"() -> (w203:dbl)
            n104 = local read "Step Size"() -> (w205:dbl)
            n105 = Number To Decimal String(number=w202) -> (decimal integer string=w210:string)  [unwired: 1 in]
            n106 = Number To Fractional String(number=w203) -> (F-format string=w220:string)  [unwired: 3 in]
            n107 = Number To Decimal String(number=w188) -> (decimal integer string=w189:string)  [unwired: 1 in]
            n108 = Number To Fractional String(number=w205) -> (F-format string=w215:string)  [unwired: 3 in]
            n109 = Number To Fractional String(number=w204) -> (F-format string=w214:string)  [unwired: 3 in]
            n110 = Concatenate Strings(w220, "\r\n", w214, "\r\n", w215, "\r\n", w210, "\r\n", w189, "\r\n", w191) -> (w218:string)
            n111 = call "File Dialog"("start path"=path "C:/Users/Raman Lab/Desktop/Molly") -> ("selected path"=w213:path)  [unwired: 11 in, 3 out]
            n112 = Write to Text File(file (use dialog)=w213, text=w218) -> ()  [unwired: 2 in, 3 out]
          }
        }
      }
      frame "Confocal Scan" {
        n113 = case shown="True" "OK Button 5" {
          tunnel: w330 -> [_ w338]
          tunnel: [_ w337] -> w329
          tunnel: [_ w336] -> _
          tunnel: w328 -> [_ w335]
          tunnel: [_ w334] -> w326
          tunnel: [_ w333] -> w325
          tunnel: w324 -> [_ w332]
          tunnel: w323 -> [_ w331]
          frame False {
          }
          frame True {
            n114 = stacked-sequence {
              seq-local: [w340 _] -> [_ w380]
              seq-local: [w339 _] -> [_ w379]
              tunnel: w338 -> [w341 w383]
              tunnel: [_ w382] -> w337
              tunnel: [_ w381] -> w336
              tunnel: w335 -> [w342 _]
              tunnel: [_ w372] -> w334
              tunnel: [_ w374] -> w333
              tunnel: w332 -> [_ w371]
              tunnel: w331 -> [_ w370]
              frame #0 {
                n115 = stacked-sequence {
                  tunnel: w342 -> [w346]
                  tunnel: w341 -> [w345]
                  tunnel: [w344] -> w339
                  tunnel: [w343] -> w340
                  frame #0 {
                    w358 = cluster{"S/N":string, "USB Search?":bool} {"S/N"="", "USB Search?"=TRUE}  # USB settings
                    w354 = u16 2 items=["RS232", "TCP/IP", "USB"] ("Interface")
                    w353 = cluster{"Portnumber":i32, "Baudrate":u16} {"Portnumber"=0, "Baudrate"=5}  # RS232 settings
                    w352 = T3 {"Host address/name"="", "Port"=50000, "Board"=0, "TCP/IP Search?"=TRUE}  # TCP/IP settings
                    # "TRUE: We want to\nmove the axis to its middle\nposition"
                    # "System number is one"
                    n116 = call "E727_Configuration_Setup.vi"("System no."=w345, "USB settings"=w358, "Are stages connected?"=bool[] [TRUE, TRUE, FALSE], "Change servo status to ON?"=TRUE ("Use dialog to define\nconnected stages?"), "Perform autozero?"=FALSE ("Use dialog to define\nconnected stages?"), "error in"=w346, "Interface"=w354, "RS232 settings"=w353, "TCP/IP settings"=w352, "Stop wave generator\noutput (if any)"=TRUE ("All axes?"), "Move to middle?"=FALSE) -> ("All conn. axes"=w343:string[], "error out"=w348:errorcluster)  [unwired: 3 in, 4 out]
                    n117 = call "POS?.vi"("System no."=w345, "Axes to query"=w343, "All axes?"=TRUE, "error in"=w348) -> ("Position"=→"Position 2":dbl[], "error out"=w344:errorcluster)  [unwired: 1 in, 13 out]
                  }
                }
              }
              frame #1 {
                n118 = for {
                  N: "Number of Steps Left" -> [w384]
                  tunnel: w383 -> [w400]
                  tunnel: [w394] -> w369 mode=indexing
                  tunnel: [w402] -> w381
                  tunnel: w380 -> [w401]
                  tunnel: w379 -> [w399]
                  tunnel: [w398] -> w382
                  tunnel: [w391] -> w373
                  tunnel: [w390] -> w375
                  tunnel: w371 -> [w386]
                  tunnel: w370 -> [w385]
                  stop <- "stop 2" stop-if-true
                  n119 = call <userlib>:"CameraShutter.vi"("Shutter Comp Time: Pre Open"=w385, "error in"=w386, "Shutter State"=3) -> ("Camera Handle"=w388:u32, "error out"=w387:errorcluster)  [unwired: 2 in]
                  n120 = Multiply(x="Step Size (microns)", y=-1) -> (x*y=w395:dbl[])
                  n121 = local write "Step Size (microns)"(w395) -> ()
                  n122 = stacked-sequence {
                    seq-local: [w409 _] -> [_ w503]
                    seq-local: [w410 _] -> [_ w505]
                    tunnel: [_ w504] -> w402
                    tunnel: w401 -> [w413 w506]
                    tunnel: w400 -> [w411 _]
                    tunnel: w399 -> [w412 _]
                    tunnel: [_ w503] -> w398
                    tunnel: [w408 _] -> w392
                    tunnel: [w407 _] -> w391
                    tunnel: [w406 _] -> w390
                    tunnel: w388 -> [w405 _]
                    tunnel: w387 -> [w404 _]
                    frame #0 {
                      n123 = while {
                        shift-right: [w435] -> w414
                        shift-left: dbl[][] [] -> [w436]
                        shift-right: [w418] -> w408
                        shift-left: dbl[][] [] -> [w419]
                        tunnel: w412 -> [w434]
                        tunnel: w413 -> [w433]
                        tunnel: w411 -> [w430]
                        tunnel: [w429] -> w410
                        tunnel: [w428] -> w409
                        tunnel: [w425] -> w407
                        tunnel: [w424] -> w406
                        tunnel: w405 -> [w423]
                        tunnel: w404 -> [w422]
                        i -> [w431]
                        stop <- w432 stop-if-true
                        n124 = Increment(x=w431) -> (x+1=w427:i32)
                        n125 = stacked-sequence {
                          tunnel: w434 -> [w453 _]
                          tunnel: [w446 _] -> w429
                          tunnel: w433 -> [w444 _]
                          tunnel: w427 -> [_ _]
                          tunnel: w430 -> [w439 _]
                          tunnel: [w439 _] -> w428
                          tunnel: [_ w458] -> w420
                          tunnel: [_ w457] -> w425
                          tunnel: [_ w456] -> w424
                          tunnel: w423 -> [_ w455]
                          tunnel: w422 -> [_ w454]
                          frame #0 {
                            # "Use first\naxis only."
                            # "Wait until move\nhas stopped or\nstop is pressed"
                            # "Move first axis 0.01 mm\nrelative to its current\nposition."
                            n126 = local read "Step Size (microns)"() -> (w438:dbl[])
                            n127 = Index Array(array=w444, index=0) -> (element=w447:string)
                            n128 = Build Array(w447) -> (w443:string[])
                            n129 = call "MOV.vi"("System no."=w439, "Axes to move"=w443, "Position values"=w438, "error in"=w453) -> ("error out"=w451:errorcluster)  [unwired: 1 in, 14 out]
                            n130 = call "General wait for movement to stop.vi"("System no."=w439, "Axes to wait for"=w443, "error in"=w451) -> ("error out"=w445:errorcluster)  [unwired: 5 in, 11 out]
                            n131 = call "POS?.vi"("System no."=w439, "Axes to query"=w443, "All axes?"=TRUE, "error in"=w445) -> ("Position"=w442:dbl[], "error out"=w450:errorcluster)  [unwired: 1 in, 13 out]
                            "Position" <- w442
                            n132 = Split 1D Array(array=w442, index=1) -> (first subarray=w440:dbl[])  [unwired: 1 out]
                            n133 = call "ERR?.vi"("System no."=w439, "error in"=w450) -> ("error out"=w449:errorcluster)  [unwired: 17 out]
                            n134 = Add Array Elements(numeric array=w440) -> ()  [unwired: 1 out]
                            n135 = call "GCSTranslateError.vi"("error in"=w449) -> ("error out"=w446:errorcluster)  [unwired: 18 out]
                          }
                          frame #1 {
                            n136 = global read "GlobalFramesToStr.vi" "Frames to Store"() -> (w466:u32)
                            n137 = call "ExSubCreateFile.vi"("error in (no error)"=w454, "Pulser Handle"=u32 0, "Camera Handle"=w455) -> ("error out"=w468:errorcluster, "Handles Out"=w464:T4)  [unwired: 1 in]
                            n138 = Unbundle(w464) -> ("File Handle"=w459:u32, "Image Handle"=w462:u32)  [unwired: 3 out]
                            n139 = call <userlib>:"CameraStart.vi"("error in"=w468) -> ("error out"=w463:errorcluster, "Camera Handle"=w461:u32)  [unwired: 1 in]
                            n140 = for {
                              N: w466 -> [_]
                              tunnel: w463 -> [w473]
                              tunnel: [w472] -> w465
                              tunnel: w459 -> [w471]
                              tunnel: w462 -> [w470]
                              tunnel: [w469] -> w458 mode=indexing
                              n141 = while {
                                tunnel: [w480] -> w472
                                tunnel: w473 -> [w478]
                                tunnel: w471 -> [w477]
                                tunnel: w470 -> [w476]
                                tunnel: [w475] -> w469
                                stop <- w481 stop-if-true
                                n142 = call <userlib>:"CameraCheckData.vi"("error in"=w478) -> ("Camera Handle"=w483:u32, "Number Of Frames Available"=w485:i32, "error out"=w482:errorcluster)  [unwired: 1 in]
                                n143 = Wait Until Next ms Multiple(millisecond multiple=u32 50) -> ()  [unwired: 1 out]
                                n144 = Greater Than 0?(x=w485) -> (x > 0?=w484:bool)
                                n145 = case shown="True" w484 {
                                selector: w484 -> [w486 w496]
                                tunnel: w483 -> [_ w498]
                                tunnel: w482 -> [w487 w497]
                                tunnel: [w486 w496] -> w481
                                tunnel: [w487 w491] -> w480
                                tunnel: w477 -> [_ w490]
                                tunnel: w476 -> [_ w489]
                                tunnel: [_ w488] -> w475
                                frame False {
                                }
                                frame True {
                                w492 = 1
                                n146 = call <userlib>:"CameraGetData.vi"("error in"=w497, "Image/Data Handle"=w489, "Camera Handle"=w498) -> ("error out"=w495:errorcluster, "Image/Data Handle"=w493:u32)  [unwired: 1 out]
                                n147 = call <userlib>:"FileSaveData.vi"("error in"=w495, "Image Handle"=w493, "File Handle"=w490) -> ("error out"=w494:errorcluster)  [unwired: 1 out]
                                n148 = call <userlib>:"ImageGetLineF32.vi"("error in"=w494, "Z Position"=w492, "Y Position"=w492, "Data Handle"=w493) -> ("error out"=w491:errorcluster, "Array F32"=w488:sgl[])  [unwired: 1 out]
                                }
                                }
                              }
                              n149 = Wait Until Next ms Multiple(millisecond multiple=u32 50) -> ()  [unwired: 1 out]
                            }
                            n150 = call <userlib>:"CameraStop.vi"("error in"=w465, "Camera Handle"=w461) -> ("error out"=w467:errorcluster, "Camera Handle"=w456:u32)
                            n151 = call "ExSubCloseFileImage.vi"("error in (no error)"=w467, "Handles In"=w464) -> ("error out"=w457:errorcluster)
                          }
                        }
                        n152 = Greater Or Equal?(x=w427, y="Number of Steps Down") -> (x >= y?=w432:bool)
                        n153 = Build Array (concatenate)(w419, w420) -> (w418:dbl[][])
                        n154 = Add Array Elements(numeric array=w420) -> (sum=w421:sgl)
                        n155 = Build Array(w421) -> (w437:sgl[])
                        n156 = Build Array (concatenate)(w436, w437) -> (w435:dbl[][])
                      }
                      n157 = call <vilib>:"Plot Helper.vi"("y matrix"=w414) -> ("2D Plotmatrix Class Obj Array out"=→"XY Plot Matrix":refnum<class "XY Plot Matrix Datatype.lvclass">[])  [unwired: 3 in, 7 out]
                    }
                    frame #1 {
                      # "Use first\naxis only."
                      # "Wait until move\nhas stopped or\nstop is pressed"
                      # "Move first axis 0.01 mm\nrelative to its current\nposition."
                      n158 = local read "Step Size (microns)"() -> (w500:dbl[])
                      n159 = Index Array(array=w506, index=1) -> (element=w511:string)
                      n160 = Build Array(w511) -> (w509:string[])
                      n161 = Absolute Value(x=w500) -> (abs(x)=w499:dbl[])
                      n162 = call "MOV.vi"("System no."=w503, "Axes to move"=w509, "Position values"=w499, "error in"=w505) -> ("error out"=w515:errorcluster)  [unwired: 1 in, 14 out]
                      n163 = call "General wait for movement to stop.vi"("System no."=w503, "Axes to wait for"=w509, "error in"=w515) -> ("error out"=w510:errorcluster)  [unwired: 5 in, 11 out]
                      n164 = call "POS?.vi"("System no."=w503, "Axes to query"=w509, "All axes?"=TRUE, "error in"=w510) -> ("Position"=w508:dbl[], "error out"=w514:errorcluster)  [unwired: 1 in, 13 out]
                      "Position 3" <- w508
                      n165 = Split 1D Array(array=w508, index=1) -> (second subarray=w501:dbl[])  [unwired: 1 out]
                      n166 = call "ERR?.vi"("System no."=w503, "error in"=w514) -> ("error out"=w513:errorcluster)  [unwired: 17 out]
                      n167 = call "GCSTranslateError.vi"("error in"=w513) -> ("error out"=w504:errorcluster)  [unwired: 18 out]
                      n168 = Split 1D Array(array=w501, index=1) -> ()  [unwired: 2 out]
                    }
                  }
                  n169 = Array To Spreadsheet String(array=w392, 3:"%f" ("format string")) -> (spreadsheet string=w394:string)  [unwired: 1 in]
                  "Line Number" <- w384
                }
                n170 = local read "Number of Steps Left"() -> (w360:dbl)
                n171 = local read "Exposure 2"() -> (w363:dbl)
                n172 = call <userlib>:"CameraShutter.vi"("Camera Handle"=w375, "error in"=w373) -> ("Camera Handle"=w374:u32, "error out"=w372:errorcluster)  [unwired: 3 in]
                n173 = call "File Dialog3"("start path"=path "C:/Users/Raman Lab/Desktop/Molly") -> ("selected path"=w376:path)  [unwired: 11 in, 3 out]
                n174 = local read "Number of Steps Down"() -> (w368:dbl)
                n175 = Number To Decimal String(number=w360) -> (decimal integer string=w359:string)  [unwired: 1 in]
                n176 = Number To Fractional String(number=w368) -> (F-format string=w367:string)  [unwired: 3 in]
                n177 = Number To Decimal String(number=w363) -> (decimal integer string=w364:string)  [unwired: 1 in]
                n178 = Concatenate Strings(w367, "\r\n", w359, "\r\n", w364, "\r\n", w369) -> (w378:string)
                n179 = Write to Text File(file (use dialog)=w376, text=w378) -> ()  [unwired: 2 in, 3 out]
              }
            }
          }
        }
      }
      frame "RF Single Frequency" {
        n180 = case shown="True" "OK Button 4" {
          tunnel: w521 -> [w523 w548]
          tunnel: [w523 w550] -> w519
          tunnel: [w522 w549] -> w518
          tunnel: w520 -> [w522 w547]
          frame False {
          }
          frame True {
            w526 = 1
            n181 = local read "Points"() -> (w543:i32)
            n182 = Initialize Array(0.0, w543, 1.0) -> (w541:dbl[][])
            n183 = for {
              N: "number of scans" -> [_]
              shift-right: [w577] -> w550
              shift-left: w548 -> [w575]
              shift-right: [w576] -> w549
              shift-left: w547 -> [w574]
              shift-right: [w554] -> _
              shift-left: w541 -> [w557]
              tunnel: [w551] -> w539 mode=indexing
              i -> [w560]
              n184 = call <userlib>:"CameraShutter.vi"("Camera Handle"=w575, "error in"=w574, "Shutter State"=3) -> ("Camera Handle"=w564:u32, "error out"=w565:errorcluster)  [unwired: 2 in]
              n185 = for {
                N: "Points" -> [_]
                shift-right: [w582] -> _
                shift-left: "Frequency" -> [w595]
                tunnel: [w597] -> w570
                tunnel: [w596] -> w569
                shift-right: [w591] -> _
                shift-left: dbl[][] [] -> [w592]
                tunnel: w565 -> [w594]
                tunnel: w564 -> [w593]
                shift-right: [w584] -> _
                shift-left: dbl[][] [] -> [w588]
                shift-right: [w585] -> w556
                shift-left: dbl[][] [] -> [w587]
                tunnel: [w584] -> w555
                shift-right: [w579] -> w552
                shift-left: dbl[][] [] -> [w580]
                i -> [w578]
                n186 = stacked-sequence {
                  tunnel: w595 -> [w599 _]
                  tunnel: [_ w607] -> w597
                  tunnel: [_ w608] -> w596
                  tunnel: [w598 _] -> w582
                  tunnel: [_ w606] -> w586
                  tunnel: w594 -> [_ w605]
                  tunnel: w593 -> [_ w604]
                  tunnel: w578 -> [w598 _]
                  frame #0 {
                    n187 = Number To Fractional String(use system decimal point (T)=FALSE, number=w599, precision (6)=7) -> (F-format string=w603:string)  [unwired: 1 in]
                    n188 = Concatenate Strings("f", w603) -> ()  [unwired: 1 out]
                  }
                  frame #1 {
                    n189 = global read "GlobalFramesToStr.vi" "Frames to Store"() -> (w616:u32)
                    n190 = call "ExSubCreateFile.vi"("error in (no error)"=w605, "Pulser Handle"=u32 0, "Camera Handle"=w604) -> ("error out"=w618:errorcluster, "Handles Out"=w614:T4)  [unwired: 1 in]
                    n191 = Unbundle(w614) -> ("File Handle"=w609:u32, "Image Handle"=w612:u32)  [unwired: 3 out]
                    n192 = call <userlib>:"CameraStart.vi"("error in"=w618) -> ("error out"=w613:errorcluster, "Camera Handle"=w611:u32)  [unwired: 1 in]
                    n193 = for {
                      N: w616 -> [_]
                      tunnel: w613 -> [w623]
                      tunnel: [w622] -> w615
                      tunnel: w609 -> [w621]
                      tunnel: w612 -> [w620]
                      tunnel: [w619] -> w606 mode=indexing
                      n194 = while {
                        tunnel: [w630] -> w622
                        tunnel: w623 -> [w628]
                        tunnel: w621 -> [w627]
                        tunnel: w620 -> [w626]
                        tunnel: [w625] -> w619
                        stop <- w631 stop-if-true
                        n195 = call <userlib>:"CameraCheckData.vi"("error in"=w628) -> ("Camera Handle"=w633:u32, "Number Of Frames Available"=w635:i32, "error out"=w632:errorcluster)  [unwired: 1 in]
                        n196 = Wait Until Next ms Multiple(millisecond multiple=u32 50) -> ()  [unwired: 1 out]
                        n197 = Greater Than 0?(x=w635) -> (x > 0?=w634:bool)
                        n198 = case shown="True" w634 {
                          selector: w634 -> [w636 w646]
                          tunnel: w633 -> [_ w648]
                          tunnel: w632 -> [w637 w647]
                          tunnel: [w636 w646] -> w631
                          tunnel: [w637 w641] -> w630
                          tunnel: w627 -> [_ w640]
                          tunnel: w626 -> [_ w639]
                          tunnel: [_ w638] -> w625
                          frame False {
                          }
                          frame True {
                            w642 = 1
                            n199 = call <userlib>:"CameraGetData.vi"("error in"=w647, "Image/Data Handle"=w639, "Camera Handle"=w648) -> ("error out"=w645:errorcluster, "Image/Data Handle"=w643:u32)  [unwired: 1 out]
                            n200 = call <userlib>:"FileSaveData.vi"("error in"=w645, "Image Handle"=w643, "File Handle"=w640) -> ("error out"=w644:errorcluster)  [unwired: 1 out]
                            n201 = call <userlib>:"ImageGetLineF32.vi"("error in"=w644, "Z Position"=w642, "Y Position"=w642, "Data Handle"=w643) -> ("error out"=w641:errorcluster, "Array F32"=w638:sgl[])  [unwired: 1 out]
                          }
                        }
                      }
                      n202 = Wait Until Next ms Multiple(millisecond multiple=u32 50) -> ()  [unwired: 1 out]
                    }
                    n203 = call <userlib>:"CameraStop.vi"("error in"=w615, "Camera Handle"=w611) -> ("error out"=w617:errorcluster, "Camera Handle"=w607:u32)
                    n204 = call "ExSubCloseFileImage.vi"("error in (no error)"=w617, "Handles In"=w614) -> ("error out"=w608:errorcluster)
                  }
                }
                n205 = Add Array Elements(numeric array=w586) -> (sum=w583:sgl)
                n206 = Insert Into Array(array=w592, new element=w586) -> (w591:dbl[][])  [unwired: 2 in]
                n207 = Build Array(w583) -> (w589:sgl[])
                n208 = Build Array(w582) -> (w590:i32[])
                n209 = Build Array(w583, w582) -> (w581:sgl[])
                n210 = Build Array (concatenate)(w587, w589) -> (w585:dbl[][])
                n211 = Build Array (concatenate)(w588, w590) -> (w584:dbl[][])
                n212 = Build Array (concatenate)(w580, w581) -> (w579:dbl[][])
                "Point #" <- w578
              }
              n213 = Add(x=1, y=w560) -> (x+y=→"Scan #":i32)
              n214 = Add(x=w557, y=w556) -> (x+y=w554:dbl[][])
              "history 2" <- w554
              n215 = call <userlib>:"CameraShutter.vi"("Camera Handle"=w570, "error in"=w569, "Shutter State"=2) -> ("Camera Handle"=w577:u32, "error out"=w576:errorcluster)  [unwired: 2 in]
              n216 = Array To Spreadsheet String(array=w552, 3:"%f" ("format string")) -> (spreadsheet string=w551:string)  [unwired: 1 in]
              n217 = call <vilib>:"Plot Helper.vi"("y matrix"=w554, "x matrix"=w555) -> ("2D Plotmatrix Class Obj Array out"=→"XY Plot Matrix 2":refnum<class "XY Plot Matrix Datatype.lvclass">[])  [unwired: 2 in, 7 out]
            }
            n218 = local read "Frequency"() -> (w536:dbl)
            n219 = local read "number of scans"() -> (w527:i32)
            n220 = local read "Points"() -> (w537:i32)
            n221 = call "File Dialog2"("start path"=path "C:/Users/Raman Lab/Desktop/Molly") -> ("selected path"=w540:path)  [unwired: 11 in, 3 out]
            n222 = Add(x=w536, y=w537) -> (x+y=w525:dbl)
            n223 = Subtract(x=w525, y=w526) -> (x-y=w524:dbl)
            n224 = Number To Fractional String(number=w526) -> (F-format string=w529:string)  [unwired: 3 in]
            n225 = Number To Decimal String(number=w527) -> (decimal integer string=w528:string)  [unwired: 1 in]
            n226 = Number To Fractional String(number=w524) -> (F-format string=w534:string)  [unwired: 3 in]
            n227 = Number To Fractional String(number=w536) -> (F-format string=w535:string)  [unwired: 3 in]
            n228 = Concatenate Strings(w535, "\r\n", w534, "\r\n", w529, "\r\n", w528, "\r\n", w539) -> (w538:string)
            n229 = Write to Text File(file (use dialog)=w540, text=w538) -> ()  [unwired: 2 in, 3 out]
          }
        }
      }
      frame "Stage Control" {
        n230 = case shown="True" "?" {
          tunnel: w649 -> [_ w691]
          tunnel: w650 -> [_ w690]
          frame False {
          }
          frame True {
            n231 = stacked-sequence {
              seq-local: [w693 _] -> [_ w713]
              seq-local: [w692 _] -> [_ w712]
              tunnel: w690 -> [w694 _]
              tunnel: w691 -> [w695 _]
              frame #0 {
                n232 = stacked-sequence {
                  tunnel: w695 -> [w699]
                  tunnel: w694 -> [w698]
                  tunnel: [w697] -> w692
                  tunnel: [w696] -> w693
                  frame #0 {
                    w711 = cluster{"S/N":string, "USB Search?":bool} {"S/N"="", "USB Search?"=TRUE}  # USB settings
                    w707 = u16 2 items=["RS232", "TCP/IP", "USB"] ("Interface")
                    w706 = cluster{"Portnumber":i32, "Baudrate":u16} {"Portnumber"=0, "Baudrate"=5}  # RS232 settings
                    w705 = T3 {"Host address/name"="", "Port"=50000, "Board"=0, "TCP/IP Search?"=TRUE}  # TCP/IP settings
                    # "TRUE: We want to\nmove the axis to its middle\nposition"
                    # "System number is one"
                    n233 = call "E727_Configuration_Setup.vi"("System no."=w698, "USB settings"=w711, "Are stages connected?"=bool[] [TRUE, TRUE, FALSE], "Change servo status to ON?"=TRUE ("Use dialog to define\nconnected stages?"), "Perform autozero?"=FALSE ("Use dialog to define\nconnected stages?"), "error in"=w699, "Interface"=w707, "RS232 settings"=w706, "TCP/IP settings"=w705, "Stop wave generator\noutput (if any)"=TRUE ("All axes?"), "Move to middle?"=FALSE) -> ("All conn. axes"=w696:string[], "error out"=w701:errorcluster)  [unwired: 3 in, 4 out]
                    n234 = call "POS?.vi"("System no."=w698, "Axes to query"=w696, "All axes?"=TRUE, "error in"=w701) -> ("Position"=→"Position 4":dbl[], "error out"=w697:errorcluster)  [unwired: 1 in, 13 out]
                  }
                }
              }
              frame #1 {
                n235 = stacked-sequence {
                  tunnel: w713 -> [w716]
                  tunnel: w712 -> [w715]
                  frame #0 {
                    w714 = 1
                    # "Use first\naxis only."
                    # "Wait until move\nhas stopped or\nstop is pressed"
                    # "Move first axis 0.01 mm\nrelative to its current\nposition."
                    n236 = local read "Step Size (microns) Y"() -> (w717:dbl[])
                    n237 = Index Array(array=w716, index=0) -> (element=w721:string)
                    n238 = Build Array(w721) -> (w719:string[])
                    n239 = call "MOV.vi"("System no."=w714, "Axes to move"=w719, "Position values"=w717, "error in"=w715) -> ("error out"=w725:errorcluster)  [unwired: 1 in, 14 out]
                    n240 = call "General wait for movement to stop.vi"("System no."=w714, "Axes to wait for"=w719, "error in"=w725) -> ("error out"=w720:errorcluster)  [unwired: 5 in, 11 out]
                    n241 = call "POS?.vi"("System no."=w714, "Axes to query"=w719, "All axes?"=TRUE, "error in"=w720) -> ("Position"=→"Position 5":dbl[], "error out"=w724:errorcluster)  [unwired: 1 in, 13 out]
                    n242 = call "ERR?.vi"("System no."=w714, "error in"=w724) -> ("error out"=w723:errorcluster)  [unwired: 17 out]
                    n243 = call "GCSTranslateError.vi"("error in"=w723) -> ()  [unwired: 19 out]
                  }
                }
              }
            }
          }
        }
        n244 = case shown="True" "?" {
          tunnel: w649 -> [_ w654]
          tunnel: w650 -> [_ w653]
          frame False {
          }
          frame True {
            n245 = stacked-sequence {
              seq-local: [w656 _] -> [_ w676]
              seq-local: [w655 _] -> [_ w675]
              tunnel: w653 -> [w657 _]
              tunnel: w654 -> [w658 _]
              frame #0 {
                n246 = stacked-sequence {
                  tunnel: w658 -> [w662]
                  tunnel: w657 -> [w661]
                  tunnel: [w660] -> w655
                  tunnel: [w659] -> w656
                  frame #0 {
                    w674 = cluster{"S/N":string, "USB Search?":bool} {"S/N"="", "USB Search?"=TRUE}  # USB settings
                    w670 = u16 2 items=["RS232", "TCP/IP", "USB"] ("Interface")
                    w669 = cluster{"Portnumber":i32, "Baudrate":u16} {"Portnumber"=0, "Baudrate"=5}  # RS232 settings
                    w668 = T3 {"Host address/name"="", "Port"=50000, "Board"=0, "TCP/IP Search?"=TRUE}  # TCP/IP settings
                    # "TRUE: We want to\nmove the axis to its middle\nposition"
                    # "System number is one"
                    n247 = call "E727_Configuration_Setup.vi"("System no."=w661, "USB settings"=w674, "Are stages connected?"=bool[] [TRUE, TRUE, FALSE], "Change servo status to ON?"=TRUE ("Use dialog to define\nconnected stages?"), "Perform autozero?"=FALSE ("Use dialog to define\nconnected stages?"), "error in"=w662, "Interface"=w670, "RS232 settings"=w669, "TCP/IP settings"=w668, "Stop wave generator\noutput (if any)"=TRUE ("All axes?"), "Move to middle?"=FALSE) -> ("All conn. axes"=w659:string[], "error out"=w664:errorcluster)  [unwired: 3 in, 4 out]
                    n248 = call "POS?.vi"("System no."=w661, "Axes to query"=w659, "All axes?"=TRUE, "error in"=w664) -> ("Position"=→"Position 7":dbl[], "error out"=w660:errorcluster)  [unwired: 1 in, 13 out]
                  }
                }
              }
              frame #1 {
                n249 = stacked-sequence {
                  tunnel: w676 -> [w679]
                  tunnel: w675 -> [w678]
                  frame #0 {
                    w677 = 1
                    # "Use first\naxis only."
                    # "Wait until move\nhas stopped or\nstop is pressed"
                    # "Move first axis 0.01 mm\nrelative to its current\nposition."
                    n250 = local read "Step Size (microns) X"() -> (w680:dbl[])
                    n251 = Index Array(array=w679, index=1) -> (element=w684:string)
                    n252 = Build Array(w684) -> (w682:string[])
                    n253 = call "MOV.vi"("System no."=w677, "Axes to move"=w682, "Position values"=w680, "error in"=w678) -> ("error out"=w688:errorcluster)  [unwired: 1 in, 14 out]
                    n254 = call "General wait for movement to stop.vi"("System no."=w677, "Axes to wait for"=w682, "error in"=w688) -> ("error out"=w683:errorcluster)  [unwired: 5 in, 11 out]
                    n255 = call "POS?.vi"("System no."=w677, "Axes to query"=w682, "All axes?"=TRUE, "error in"=w683) -> ("Position"=→"Position 8":dbl[], "error out"=w687:errorcluster)  [unwired: 1 in, 13 out]
                    n256 = call "ERR?.vi"("System no."=w677, "error in"=w687) -> ("error out"=w686:errorcluster)  [unwired: 17 out]
                    n257 = call "GCSTranslateError.vi"("error in"=w686) -> ()  [unwired: 19 out]
                  }
                }
              }
            }
          }
        }
      }
    }
    n258 = global read "GlobalCamOpen.vi" "Camera Opened"() -> (w23:u32)
    n259 = Not(x="Release Camera") -> (.not. x?=w16:bool)
    n260 = Greater Than 0?(x=w23) -> (x > 0?=w22:bool)
    n261 = And(x=w16, y=w22) -> (x .and. y?=→"Camera Opened":bool)
    n262 = Wait Until Next ms Multiple(millisecond multiple=5) -> ()  [unwired: 1 out]
  }
  n263 = call <userlib>:"CameraClose.vi"("error in"=w8, "Camera Handle"=w5) -> ("error out"=w7:errorcluster)
  n264 = call "Close connection if open.vi"("System no."=w1) -> ("error out"=→"error out 2":errorcluster)  [unwired: 2 in, 16 out]
  n265 = call <userlib>:"UninitToolkit.vi"("error in"=w7) -> ("error out"=→"error out":errorcluster)
